vi "mod_Modulate AM.vi"   [LabVIEW 2020, in "niAMT.lvlib"]
uses:
  <vilib>/addons/Modulation/niAMT.lvlib
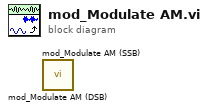
[diagram p0: block diagram]
diagram:
  n1 = call <vilib>:"mod_Modulate AM (DSB).vi"() -> ()  [unwired: 14 in, 2 out]
  n2 = call <vilib>:"mod_Modulate AM (SSB).vi"() -> ()  [unwired: 14 in, 2 out]
